vi "Show.vi"(4 "device ID":refnum<k1>, 6 "screens":T7[](array[typedef]), 8 "error in (no error)":errorcluster, 10 "TipPanel":refnum<class "TipPanel.lvclass">, 11 "loop data in":T1) -> (0 "error out":errorcluster, 3 "loop data out":T1)   [LabVIEW 2021, in "TipStripOOPanel.lvlib"]
uses:
  TipStripOOPanel.lvlib
  tipstrip_screens.ctl
  Loop Data Parent.ctl
  Classes/TipPanel/TipPanel.lvclass
  <vilib>/IlluminatedG/IG OOPanel/OOPanel/Manager/Manager.lvclass
  PanelMap.ctl
  PanelMapData.ctl
  Classes/TipPanel/ToPanelUEWrapper.ctl
  Classes/TipPanel/ToPanelUE.ctl
  <vilib>/Futures/Futures/Promise/Promise.lvclass
  refs.ctl
  content size.ctl
  <vilib>/Utility/miscctls.llb/LVRectTypeDef.ctl
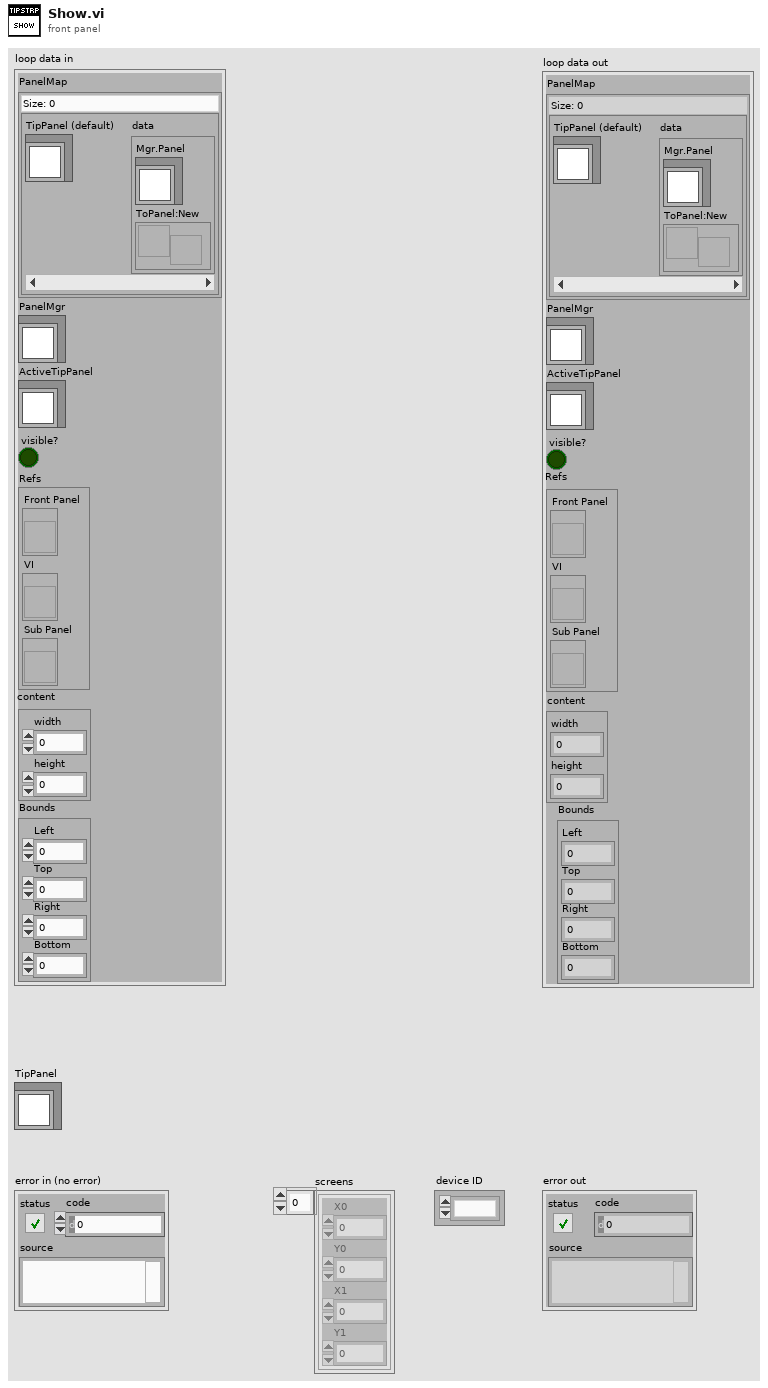
[diagram p1: front panel]
types:
  T1 = typedef "TipStripOOPanel.lvlib/Loop Data Parent.ctl" = cluster{"PanelMap":T2, "PanelMgr":refnum<class "Manager.lvclass">, "ActiveTipPanel":refnum<class "TipPanel.lvclass">, "visible?":bool, "Refs":T4, "content":T5, "Bounds":T6}
  T2 = typedef "TipStripOOPanel.lvlib/PanelMap.ctl" = map{refnum<class "TipPanel.lvclass">, T3}
  T3 = typedef "TipStripOOPanel.lvlib/PanelMapData.ctl" = cluster{"Mgr.Panel":refnum<class "TipPanel.lvclass">, "ToPanel:New":refnum<user-event>}
  T4 = typedef "TipStripOOPanel.lvlib/refs.ctl" = cluster{"Front Panel":refnum<vi>, "VI":refnum<vi>, "Sub Panel":refnum<vi>}
  T5 = typedef "TipStripOOPanel.lvlib/content size.ctl" = cluster{"width":i32, "height":i32}
  T6 = typedef "LVRectTypeDef.ctl" = cluster{"Left":i16, "Top":i16, "Right":i16, "Bottom":i16}
  T7 = typedef "TipStripOOPanel.lvlib/tipstrip_screens.ctl" = cluster{"X0":i32, "Y0":i32, "X1":i32, "Y1":i32}
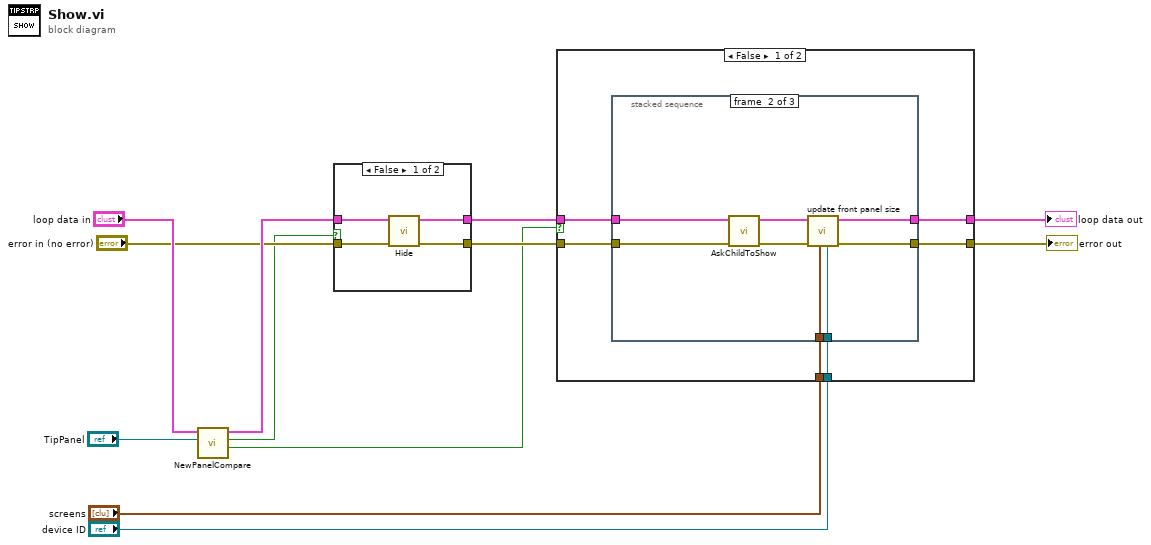
[diagram p0: block diagram]
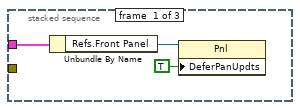
[diagram p2: hidden frame]
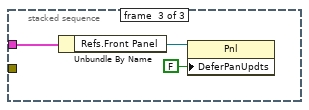
[diagram p3: hidden frame]
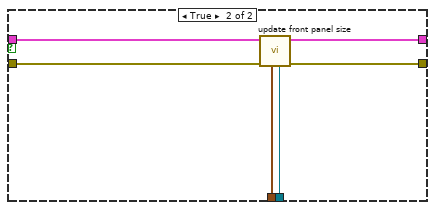
[diagram p4: hidden frame]
diagram:
  n1 = call "NewPanelCompare.vi"("TipPanel"="TipPanel", "loop data in"="loop data in") -> ("Same exact Panel?"=w5:bool, "Same Panel Type?"=w6:bool, "loop data out"=w10:T1)  [unwired: 7 in]
  n2 = case shown="False" w6 {
    tunnel: w10 -> [w16 w18]
    tunnel: [w15 w18] -> w9
    tunnel: "error in (no error)" -> [w14 w17]
    tunnel: [w13 w17] -> w7
    frame False {
      n3 = call "Hide.vi"("error in (no error)"=w14, "loop data in"=w16) -> ("error out"=w13:errorcluster, "loop data out"=w15:T1)  [unwired: 8 in]
    }
    frame True {
    }
  }
  n4 = case shown="False" w5 {
    tunnel: w9 -> [w24 w44]
    tunnel: [w23 w42] -> w2
    tunnel: w7 -> [w22 w43]
    tunnel: [w21 w41] -> w1
    tunnel: "screens" -> [w20 w40]
    tunnel: "device ID" -> [w19 w39]
    frame False {
      n5 = stacked-sequence {
        tunnel: w24 -> [w27 w35 w36]
        tunnel: [_ w31 _] -> w23
        tunnel: w22 -> [_ w34 _]
        tunnel: [_ w30 _] -> w21
        tunnel: w20 -> [_ w29 _]
        tunnel: w19 -> [_ w28 _]
        frame #0 {
          n6 = Unbundle By Name(w27) -> ("Refs.Front Panel"=w26:refnum<vi>)
          n7 = property class="Pnl"(reference=w26, "DeferPanUpdts"=TRUE ("Defer Panel Updates")) -> ()  [unwired: 1 in, 2 out]
        }
        frame #1 {
          n8 = call "AskChildToShow.vi"("error in (no error)"=w34, "loop data in"=w35) -> ("error out"=w32:errorcluster, "loop data out"=w33:T1)  [unwired: 8 in]
          n9 = call "update front panel size.vi"("device ID"=w28, "screens"=w29, "error in (no error)"=w32, "loop data in"=w33) -> ("error out"=w30:errorcluster, "loop data out"=w31:T1)  [unwired: 6 in]
        }
        frame #2 {
          n10 = Unbundle By Name(w36) -> ("Refs.Front Panel"=w38:refnum<vi>)
          n11 = property class="Pnl"(reference=w38, "DeferPanUpdts"=FALSE ("Defer Panel Updates")) -> ()  [unwired: 1 in, 2 out]
        }
      }
    }
    frame True {
      n12 = call "update front panel size.vi"("device ID"=w39, "screens"=w40, "error in (no error)"=w43, "loop data in"=w44) -> ("error out"=w41:errorcluster, "loop data out"=w42:T1)  [unwired: 6 in]
    }
  }
  "error out" <- w1
  "loop data out" <- w2
